vi "AB_860_900_Project_App_Info.vi"(7 "action":T1, 8 "error in (no error)":errorcluster, 10 "applicationInfo in":T2, 11 "Object In":T3) -> (0 "error out":errorcluster, 2 "Application info":T2, 3 "Object Out":T3)   [LabVIEW 2020]
uses:
  <resource>/Framework/Providers/API/ItemRef.ctl
  <vilib>/AppBuilder/RW_Project/AB_RW_Project_PropBag_Action.ctl
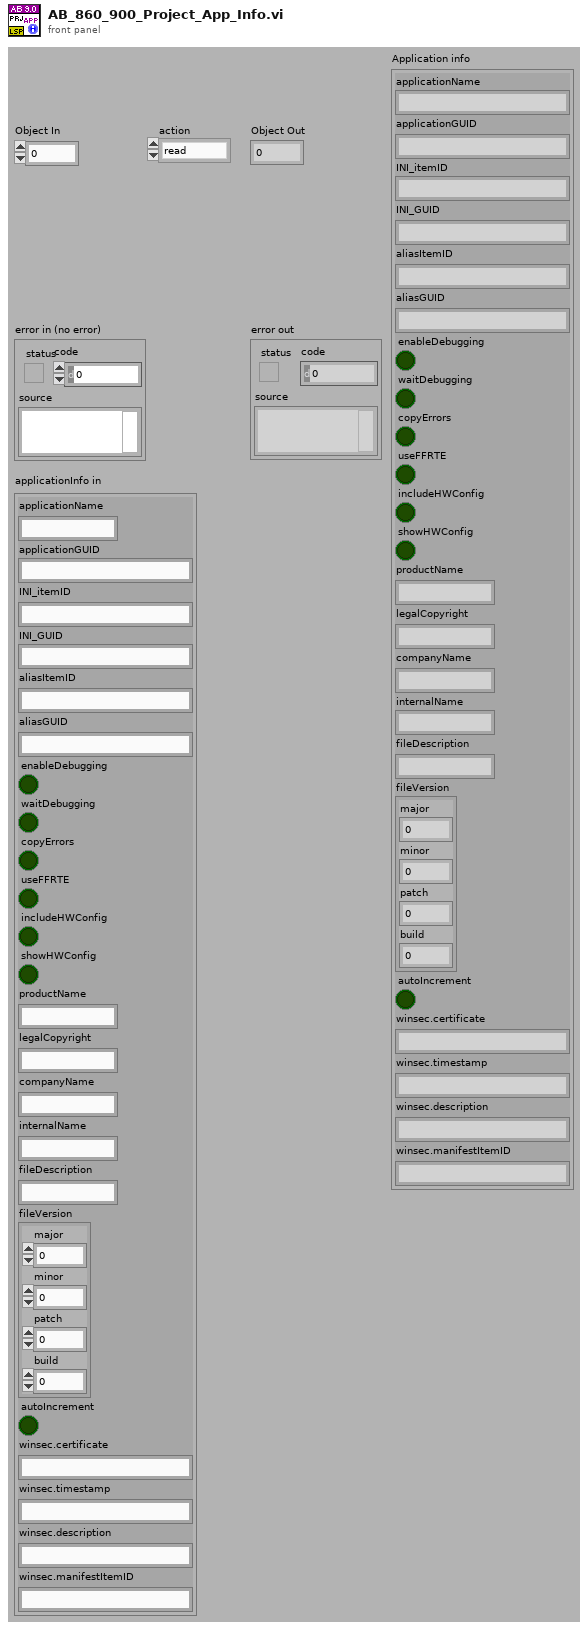
[diagram p1: front panel]
types:
  T1 = typedef "AB_RW_Project_PropBag_Action.ctl" = enum16{"read", "write", "clear", "readPrevious", "writePrevious", "clearPrevious"}
  T2 = cluster{"applicationName":string, "applicationGUID":string, "INI_itemID":string, "INI_GUID":string, "aliasItemID":string, "aliasGUID":string, "enableDebugging":bool, "waitDebugging":bool, "copyErrors":bool, "useFFRTE":bool, "includeHWConfig":bool, "showHWConfig":bool, "productName":string, "legalCopyright":string, "companyName":string, "internalName":string, "fileDescription":string, "fileVersion":cluster{"major":u16, "minor":u16, "patch":u16, "build":u16}, "autoIncrement":bool, "winsec.certificate":string, "winsec.timestamp":string, "winsec.description":string, "winsec.manifestItemID":string}
  T3 = typedef "ItemRef.ctl" = u64
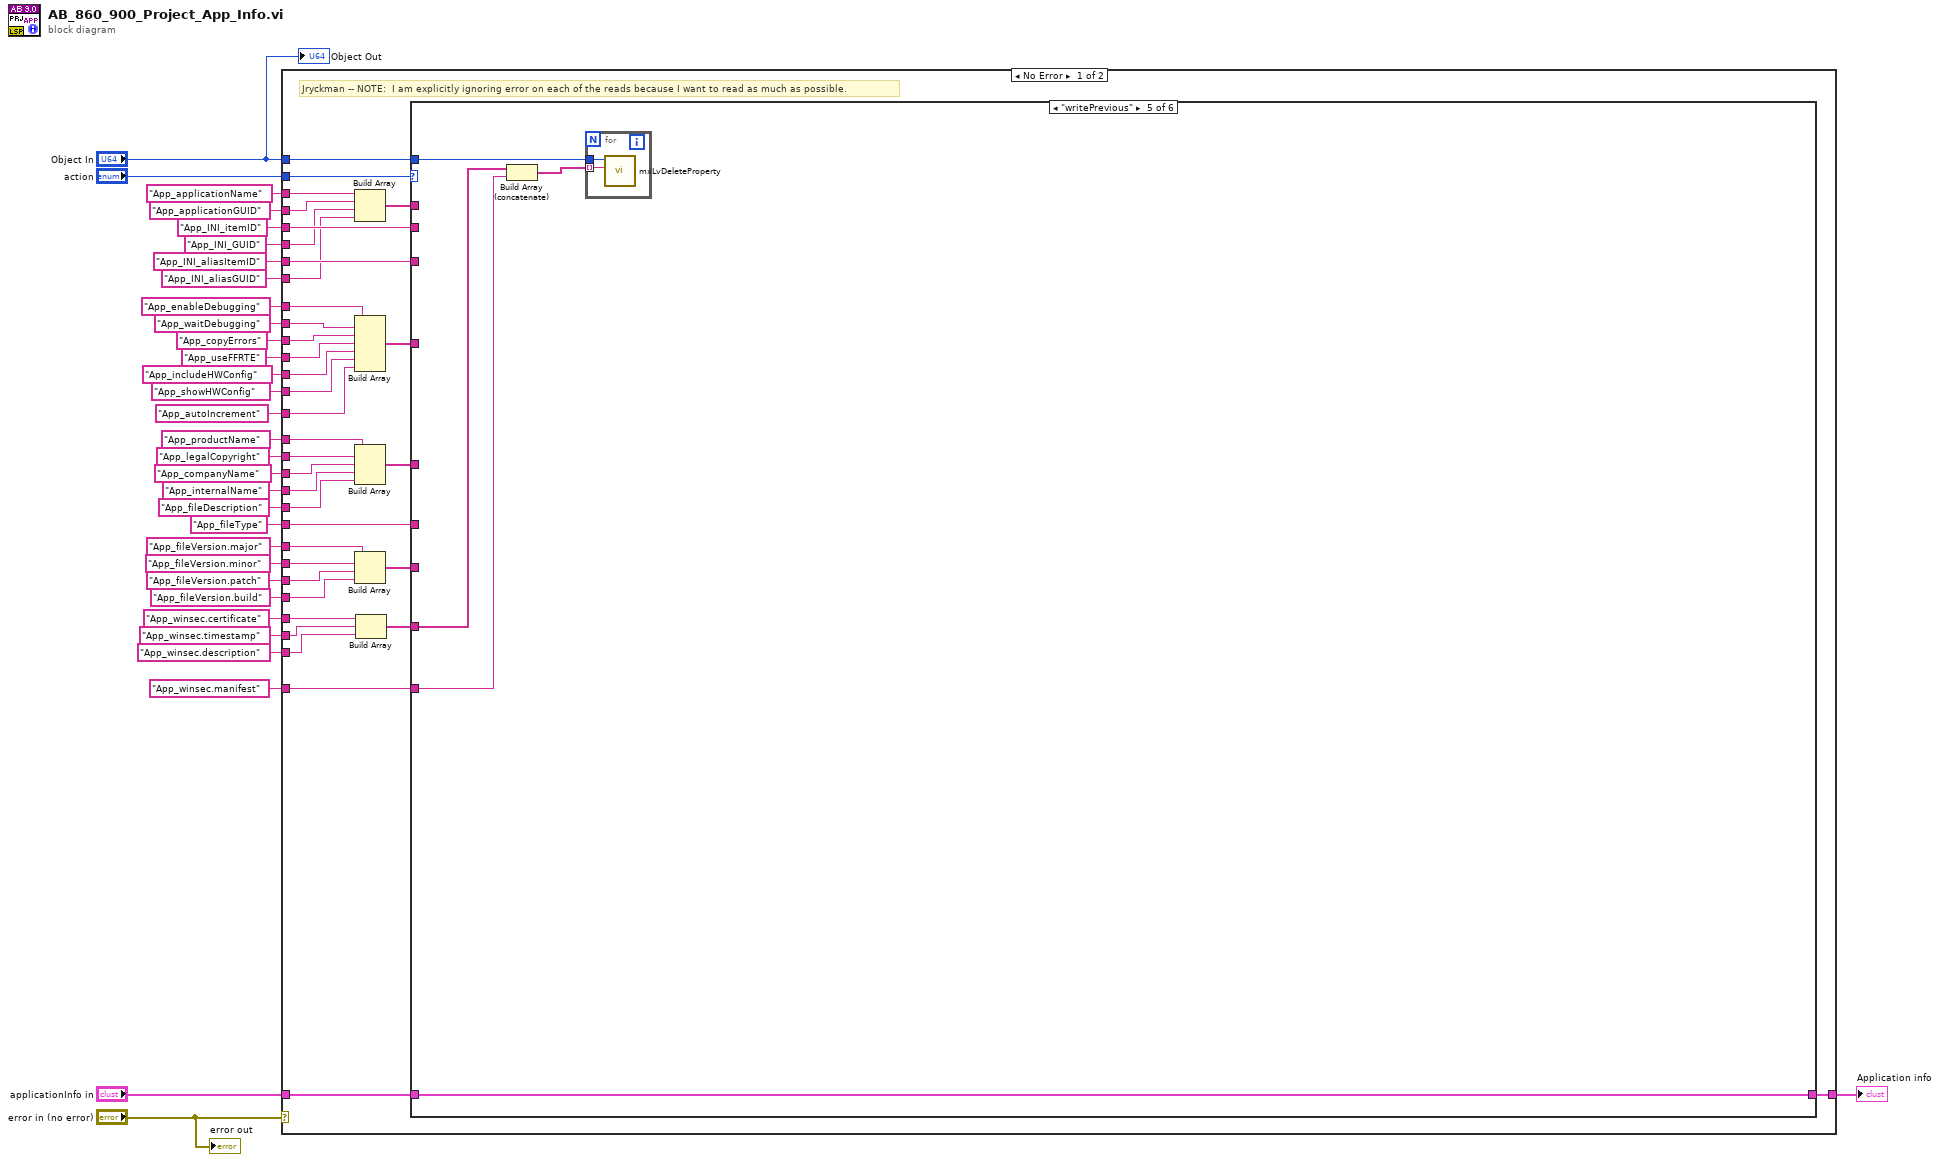
[diagram p0: block diagram]
diagram:
  n1 = case shown="No Error" "error in (no error)" {
    tunnel: "Object In" -> [w68 _]
    tunnel: [w45 _] -> w30
    tunnel: "applicationInfo in" -> [w51 _]
    tunnel: "App_applicationName" ("Tag") -> [w42 _]
    tunnel: "App_INI_itemID" ("Tag") -> [w67 _]
    tunnel: "App_INI_aliasItemID" ("Tag") -> [w66 _]
    tunnel: "App_enableDebugging" ("Tag") -> [w65 _]
    tunnel: "App_waitDebugging" ("Tag") -> [w64 _]
    tunnel: "App_copyErrors" ("Tag") -> [w63 _]
    tunnel: "App_useFFRTE" ("Tag") -> [w62 _]
    tunnel: "App_includeHWConfig" ("Tag") -> [w61 _]
    tunnel: "App_showHWConfig" ("Tag") -> [w60 _]
    tunnel: "App_productName" ("Tag") -> [w56 _]
    tunnel: "App_legalCopyright" ("Tag") -> [w57 _]
    tunnel: "App_companyName" ("Tag") -> [w55 _]
    tunnel: "App_internalName" ("Tag") -> [w54 _]
    tunnel: "App_fileDescription" ("Tag") -> [w53 _]
    tunnel: "App_fileType" ("Tag") -> [w43 _]
    tunnel: "App_fileVersion.major" ("Tag") -> [w49 _]
    tunnel: "App_fileVersion.minor" ("Tag") -> [w50 _]
    tunnel: "App_fileVersion.patch" ("Tag") -> [w48 _]
    tunnel: "App_fileVersion.build" ("Tag") -> [w47 _]
    tunnel: "App_autoIncrement" ("Tag") -> [w59 _]
    tunnel: "action" -> [w44 _]
    tunnel: "App_applicationGUID" ("Tag") -> [w41 _]
    tunnel: "App_INI_GUID" ("Tag") -> [w40 _]
    tunnel: "App_INI_aliasGUID" ("Tag") -> [w39 _]
    tunnel: "App_winsec.certificate" ("Tag") -> [w37 _]
    tunnel: "App_winsec.timestamp" ("Tag") -> [w36 _]
    tunnel: "App_winsec.description" ("Tag") -> [w35 _]
    tunnel: "App_winsec.manifest" ("Tag") -> [w33 _]
    frame No Error {
      # "Jryckman -- NOTE:  I am explicitly ignoring error on each of the reads because I want to read as much as possible."
      n2 = Build Array(w42, w41, w40, w39) -> (w38:string[])
      n3 = Build Array(w65, w64, w63, w62, w61, w60, w59) -> (w58:string[])
      n4 = Build Array(w56, w57, w55, w54, w53) -> (w52:string[])
      n5 = Build Array(w49, w50, w48, w47) -> (w46:string[])
      n6 = Build Array(w37, w36, w35) -> (w34:string[])
      n7 = case shown="\"writePrevious\"" w44 {
        tunnel: w68 -> [_ _ _ _ w76 _]
        tunnel: w67 -> [_ _ _ _ _ _]
        tunnel: w66 -> [_ _ _ _ _ _]
        tunnel: w58 -> [_ _ _ _ _ _]
        tunnel: w52 -> [_ _ _ _ _ _]
        tunnel: w51 -> [w69 w70 w71 w72 w77 w80]
        tunnel: w46 -> [_ _ _ _ _ _]
        tunnel: [w69 w70 w71 w72 w77 w80] -> w45
        tunnel: w43 -> [_ _ _ _ _ _]
        tunnel: w38 -> [_ _ _ _ _ _]
        tunnel: w34 -> [_ _ _ _ w74 _]
        tunnel: w33 -> [_ _ _ _ w75 _]
        frame "read" {
        }
        frame "write" {
        }
        frame "clear" {
        }
        frame "readPrevious" {
        }
        frame "writePrevious" {
          n8 = Build Array (concatenate)(w74, w75) -> (w73:string[])
          n9 = for {
            tunnel: w76 -> [w79]
            tunnel: w73 -> [w78] mode=indexing
            n10 = call <resource>:"mxLvDeleteProperty.vi"("Tag"=w78, "Item"=w79) -> ()  [unwired: 1 in, 9 out]
          }
        }
        frame "clearPrevious" {
        }
      }
    }
    frame Error {
    }
  }
  "Application info" <- w30
  "Object Out" <- "Object In"
  "error out" <- "error in (no error)"
